vi "trash_Parse Info Log.vi"(10 "Index Timestamp":u64=1724348542139323000, 11 "Error Log":string) -> (3 "Filtered Config Entries":string)   [LabVIEW 2021]
uses:
  CIFLogs.lvlib
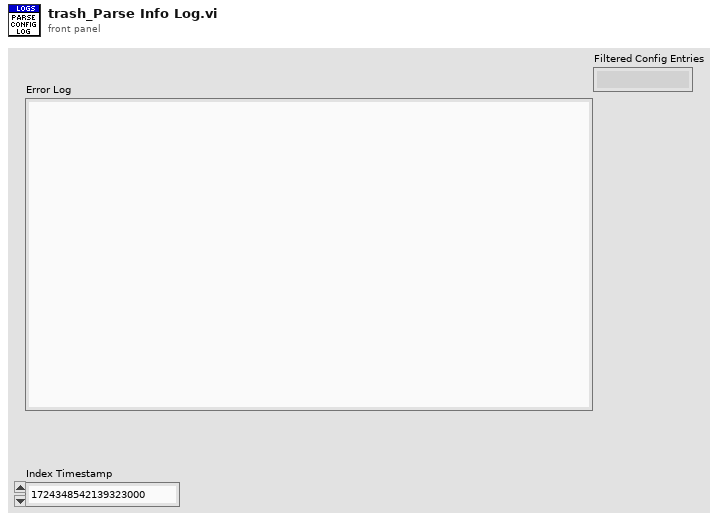
[diagram p1: front panel]
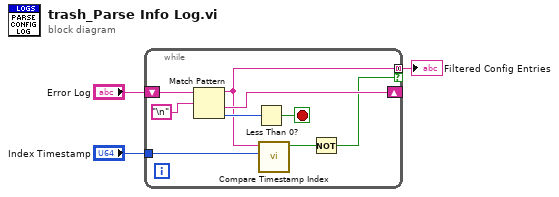
[diagram p0: block diagram]
diagram:
  n1 = while {
    shift-right: [w10] -> _
    shift-left: "Error Log" -> [w12]
    tunnel: "Index Timestamp" -> [w7]
    tunnel: [w6] -> w1 mode=concatenating if=w4
    stop <- w8 stop-if-true
    n2 = Match Pattern(string=w12, regular expression="\n") -> (before substring=w6:string, after substring=w10:string, offset past match=w9:i32)  [unwired: 1 in, 1 out]
    n3 = Less Than 0?(x=w9) -> (x < 0?=w8:bool)
    n4 = call "Compare Timestamp Index.vi"("Index Timestamp"=w7, "Log Timestamp"=w6) -> ("Past"=w5:bool)  [unwired: 9 in]
    n5 = Not(x=w5) -> (.not. x?=w4:bool)
  }
  "Filtered Config Entries" <- w1
